vi "Register Events.vi"(8 "error in (no error)":errorcluster, 11 "Software Lock-in in":refnum<class "Software Lock-in.lvclass">) -> (0 "error out":errorcluster, 1 "Output Events":refnum<event-registration>, 2 "Input Events":refnum<event-registration>, 3 "Software Lock-in out":refnum<class "Software Lock-in.lvclass">)   [LabVIEW 2015, in "Software Lock-in.lvclass"]
uses:
  Software Lock-in.lvclass
  Mag Lab Root/Mag Lab Root.lvclass/Mag Lab Root.ctl
  Software Lock-in.lvclass/Software Lock-in.ctl
  Mag Lab Root/Mag Lab Root.lvclass
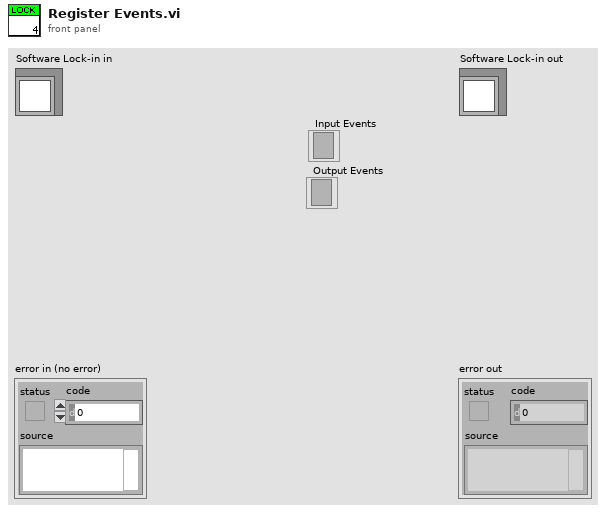
[diagram p1: front panel]
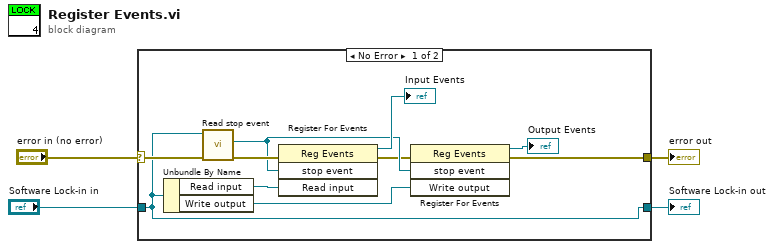
[diagram p0: block diagram]
diagram:
  n1 = case shown="No Error" "error in (no error)" {
    selector: "error in (no error)" -> [w14 w16]
    tunnel: [w6 w16] -> w3
    tunnel: [w13 w15] -> w1
    tunnel: "Software Lock-in in" -> [w13 w15]
    frame No Error {
      n2 = Unbundle By Name(w13) -> ("Read input"=w12:refnum<user-event>, "Write output"=w8:refnum<user-event>)
      n3 = call "Read stop event.vi"("error in (no error)"=w14, "Mag Lab Root in"=w13) -> ("error out"=w11:errorcluster, "stop event"=w9:refnum<user-event>)  [unwired: 7 in, 1 out]
      n4 = register-events(error in=w11, w9, w12) -> (reference out=→"Input Events":refnum<event-registration>, error out=w7:errorcluster)  [unwired: 1 in]
      n5 = register-events(error in=w7, w9, w8) -> (reference out=→"Output Events":refnum<event-registration>, error out=w6:errorcluster)  [unwired: 1 in]
    }
    frame Error {
    }
  }
  "error out" <- w3
  "Software Lock-in out" <- w1
